vi "Read reset.vi"(8 "error in (no error)":errorcluster, 11 "niUSRP Sync v1 FPGA in":refnum<class "niUSRP Sync v1 FPGA.lvclass">) -> (0 "error out":errorcluster, 2 "reset":refnum<k21>, 3 "niUSRP Sync v1 FPGA out":refnum<class "niUSRP Sync v1 FPGA.lvclass">)   [LabVIEW 2025, in "niUSRP Sync v1 FPGA.lvclass"]
uses:
  niUSRP Rx Core v1 FPGA/niUSRP Sync v1 FPGA.lvclass
  niUSRP Rx Core v1 FPGA/niUSRP Sync v1 FPGA.lvclass/niUSRP Sync v1 FPGA.ctl
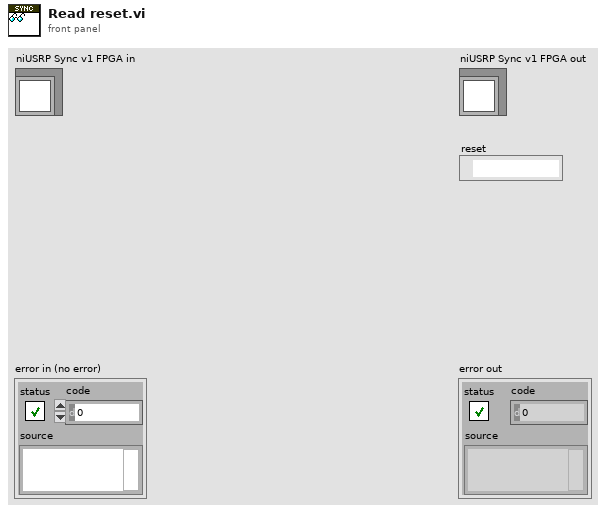
[diagram p1: front panel]
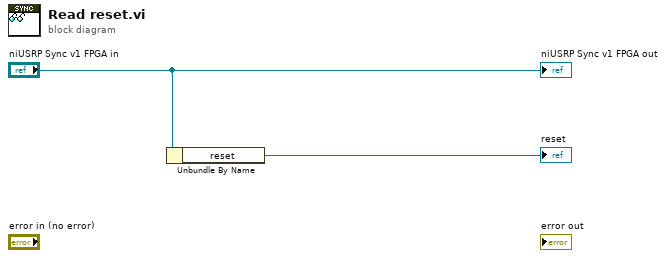
[diagram p0: block diagram]
diagram:
  n1 = Unbundle By Name("niUSRP Sync v1 FPGA in") -> ("reset"=→"reset":refnum<k21>)
  "niUSRP Sync v1 FPGA out" <- "niUSRP Sync v1 FPGA in"
